vi "Gui_SetupTrappingRF.vi"(8 "error in (no error)":errorcluster, 11 "Variant":variant) -> (0 "error out":errorcluster caption="sortie d'erreur", 3 "Variant Output":variant)   [LabVIEW 2024]
uses:
  controls/SEQUENCE_Inputs.ctl
  controls/EXCIT_Inputs.ctl
  controls/DATA_Inputs.ctl
  controls/TIMING_Inputs.ctl
  controls/PROCESSING_Inputs.ctl
  controls/TRAPPING_Inputs.ctl
  controls/RF_TRAPPING_Inputs.ctl
panel:
  in  "RF_TRAPPING Inputs":T1={"Init Values"=[0.0, 1.0, 1.0, 0.0], "Opening Values"=[0.0, -4.0, 1.0, 0.0], "Trapping Values"=[0.0, 1.0, 1.0, 0.0], "Emptying Values"=[0.0, 1.0, -7.0, 0.0], "RF Trap ON"=FALSE, "RF Accums"=1, "Number of Voltages"=4} {"RF Accums" min=1 max=100; "Trapping Values" min=-10.0 max=10.0; "Init Values" min=-10.0 max=10.0; "Emptying Values" min=-10.0 max=10.0; "Opening Values" min=-10.0 max=10.0}
  in  "CANCEL":bool
  in  "OK":bool
  in  "SEQUENCE Inputs":T2={"EXCIT Inputs"={"Number of Excitations"=1, "Script Text"="", "Table of Waveforms"=[]}, "DATA Inputs"={"Record Length"=8192, "Sample Rate"=4.0, "Data Type"=0, "Vertical Range"=0.0, "Acquisition Duration"=100000.0}, "TIMING Inputs"={"Number of Acquisitions "=1, "Number of Accumulations"=1, "Table of Waveforms"=[], "Script Text"=""}, "PROCESSING Inputs"={"Reference Mass"=300.0939, "Cyclotron Freq"=255.727, "Magnetron Freq"=0.001}, "TRAPPING Inputs"={"Number of Channels"=4, "Init Values"=[2.0, 5.0, 5.0, 2.0], "Opening Values"=[0.0, 0.0, 0.0, 0.0], "Trapping Values"=[2.0, 5.0, 5.0, 2.0], "Emptying Values"=[-5.0, -5.0, -5.0, -5.0], "Adiabatic ON"=FALSE, "Adiabatic Duration"=0, "Adiabatic Waveforms"=["Adiabatic_None_2_2_2000.bin", "Adiabatic_Ramp_5_0_2000.bin", "Adiabatic_DoubleRamp_5_0_2000.bin", "Adiabatic_RC_2_0_2000.bin"], "Ions Refill ON"=FALSE, "Number of Ions Refills"=4}, "RF_TRAPPING Inputs"={"Init Values"=[0.0, 1.0, 1.0, 0.0], "Opening Values"=[0.0, -4.0, 1.0, 0.0], "Trapping Values"=[0.0, 1.0, 1.0, 0.0], "Emptying Values"=[0.0, 1.0, -7.0, 0.0], "RF Trap ON"=FALSE, "RF Accums"=1, "Number of Voltages"=4}} {"RF_TRAPPING Inputs"."RF Accums" min=1 max=100; "RF_TRAPPING Inputs"."Trapping Values" min=-10.0 max=10.0; "RF_TRAPPING Inputs"."Init Values" min=-10.0 max=10.0; "RF_TRAPPING Inputs"."Emptying Values" min=-10.0 max=10.0; "RF_TRAPPING Inputs"."Opening Values" min=-10.0 max=10.0; "TRAPPING Inputs"."Number of Ions Refills" min=1 max=1000; "TRAPPING Inputs"."Trapping Values" min=-10.0 max=10.0; "TRAPPING Inputs"."Init Values" min=-10.0 max=10.0; "TRAPPING Inputs"."Emptying Values" min=-10.0 max=10.0; "TRAPPING Inputs"."Opening Values" min=-10.0 max=10.0; "PROCESSING Inputs"."Magnetron Freq" format="%.5g"; "PROCESSING Inputs"."Cyclotron Freq" format="%.5g"; "PROCESSING Inputs"."Reference Mass" format="%.5g"; "TIMING Inputs"."Number of Accumulations" min=0 max=50 step=1; "TIMING Inputs"."Number of Acquisitions" min=1 max=10 step=1; "DATA Inputs"."Vertical Range" items=["0.2"=0.2, "0.4"=0.4, "1"=1.0, "2"=2.0, "4"=4.0, "10"=10.0]; "DATA Inputs"."Data Type" items=["I16", "DBL"]; "DATA Inputs"."Sample Rate" items=["1 MHz"=1000000.0, "2 MHz"=2000000.0, "5 MHz"=5000000.0, "10 MHz"=10000000.0, "20 MHz"=20000000.0, "25 MHz"=25000000.0, "50 MHz"=50000000.0, "100 MHz"=100000000.0]; "EXCIT Inputs"."Number of Excitations" min=1 max=10}
  # "RF_V1"
  # "RF_V2"
  # "RF_V3"
  # "RF_V4"
  # "RF_V1"
  # "RF_V2"
  # "RF_V3"
  # "RF_V4"
  # "GO_out"
  # "Gout"
  # "GI_in"
  # "Gin"
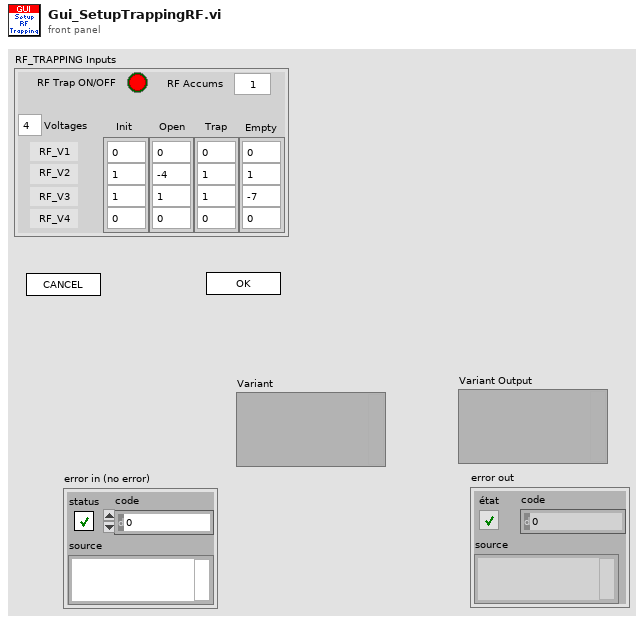
[diagram p1: front panel]
types:
  T1 = typedef "RF_TRAPPING_Inputs.ctl" = cluster{"Init Values":dbl[], "Opening Values":dbl[], "Trapping Values":dbl[], "Emptying Values":dbl[], "RF Trap ON":bool, "RF Accums":i32, "Number of Voltages":i32}
  T2 = typedef "SEQUENCE_Inputs.ctl" = cluster{"EXCIT Inputs":T3, "DATA Inputs":T4, "TIMING Inputs":T5, "PROCESSING Inputs":T6, "TRAPPING Inputs":T7, "RF_TRAPPING Inputs":T1}
  T3 = typedef "EXCIT_Inputs.ctl" = cluster{"Number of Excitations":i32, "Script Text":string, "Table of Waveforms":string[]}
  T4 = typedef "DATA_Inputs.ctl" = cluster{"Record Length":i32, "Sample Rate":dbl, "Data Type":u8, "Vertical Range":dbl, "Acquisition Duration":dbl}
  T5 = typedef "TIMING_Inputs.ctl" = cluster{"Number of Acquisitions ":i16, "Number of Accumulations":i16, "Table of Waveforms":string[], "Script Text":string}
  T6 = typedef "PROCESSING_Inputs.ctl" = cluster{"Reference Mass":dbl, "Cyclotron Freq":dbl, "Magnetron Freq":dbl}
  T7 = typedef "TRAPPING_Inputs.ctl" = cluster{"Number of Channels":i32, "Init Values":dbl[], "Opening Values":dbl[], "Trapping Values":dbl[], "Emptying Values":dbl[], "Adiabatic ON":bool, "Adiabatic Duration":i32, "Adiabatic Waveforms":string[], "Ions Refill ON":bool, "Number of Ions Refills":i32}
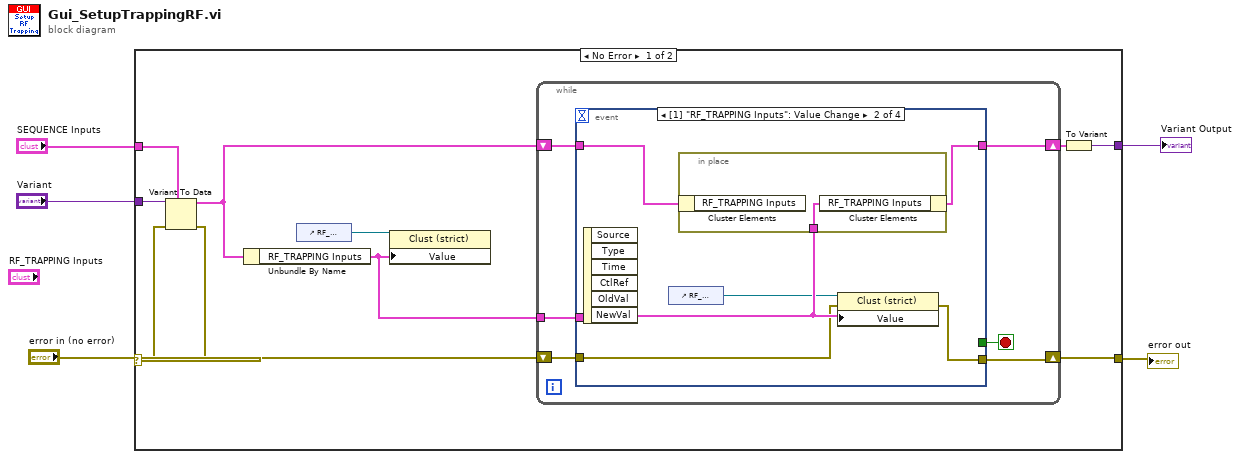
[diagram p0: block diagram]
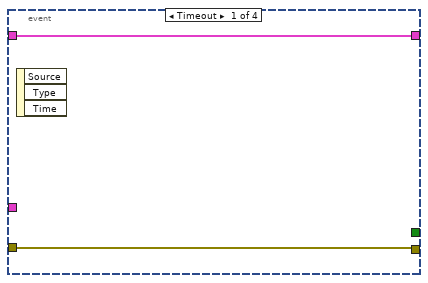
[diagram p2: hidden frame]
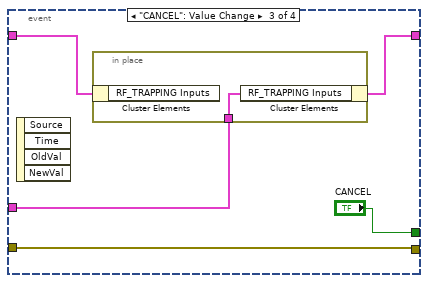
[diagram p3: hidden frame]
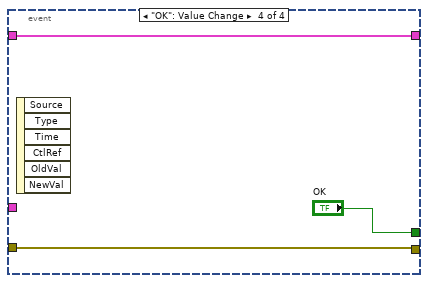
[diagram p4: hidden frame]
diagram:
  n1 = case shown="No Error" "error in (no error)" {
    selector: "error in (no error)" -> [w12 w41]
    tunnel: [w15 w41] -> w4
    tunnel: "Variant" -> [w14 w40]
    tunnel: [w7 w40] -> w2
    tunnel: "SEQUENCE Inputs" -> [w10 _]
    frame No Error {
      n2 = Variant To Data(error in=w12, type=w10, Variant=w14) -> (data=w13:T2, error out=w11:errorcluster)
      n3 = Unbundle By Name(w13) -> ("RF_TRAPPING Inputs"=w8:T1)
      n4 = control-ref of="RF_TRAPPING Inputs"() -> (w6:refnum<vi>)
      n5 = property class="Clust (strict)"(reference=w6, "Value"=w8) -> ()  [unwired: 1 in, 2 out]
      n6 = while {
        shift-right: [w18] -> w15
        shift-left: w11 -> [w19]
        shift-right: [w20] -> w9
        shift-left: w13 -> [w21]
        tunnel: w8 -> [w16]
        stop <- w17 stop-if-true
        n7 = event shown="[1] \"RF_TRAPPING Inputs\": Value Change" {
          selector: _ -> [_ _ _ _]
          dyn-events: _ -> [_ _ _ _]
          timeout: _ -> [_ _ _ _]
          tunnel: w21 -> [w23 w29 w35 w38]
          tunnel: [w23 w28 w34 w38] -> w20
          tunnel: w19 -> [w22 w25 w31 w39]
          tunnel: [w22 w26 w31 w39] -> w18
          tunnel: [_ _ "CANCEL" "OK"] -> w17
          tunnel: w16 -> [_ _ w33 _]
          event Timeout {
            n8 = event-data() -> ()  [unwired: 1 in, 3 out]
          }
          event Value Change {
            n9 = event-data() -> ("NewVal"=w27:T1)  [unwired: 1 in, 5 out]
            n10 = control-ref of="RF_TRAPPING Inputs"() -> (w24:refnum<vi>)
            n11 = in-place {
              in-place-border: w27 -> [w30]
              n12 = in-place-cluster #1(w29) -> ()  [unwired: 1 out]
              n13 = in-place-cluster #1("RF_TRAPPING Inputs"=w30) -> (w28:T2)
            }
            n14 = property class="Clust (strict)"(reference=w24, error in=w25, "Value"=w27) -> (error out=w26:errorcluster)  [unwired: 1 out]
          }
          event "CANCEL": Value Change {
            n15 = event-data() -> ()  [unwired: 1 in, 4 out]
            n16 = in-place {
              in-place-border: w33 -> [w36]
              n17 = in-place-cluster #2(w35) -> ()  [unwired: 1 out]
              n18 = in-place-cluster #2("RF_TRAPPING Inputs"=w36) -> (w34:T2)
            }
          }
          event "OK": Value Change {
            n19 = event-data() -> ()  [unwired: 1 in, 6 out]
          }
        }
      }
      n20 = To Variant(anything=w9) -> (Variant=w7:variant)
    }
    frame Error {
    }
  }
  "error out" <- w4
  "Variant Output" <- w2
